vi "EndScript.vi"(8 "error in (no error)":errorcluster, 11 "VISA Refnum in":refnum<visa-resource-name>) -> (0 "error out":errorcluster, 2 "Tx for stopping code":string, 3 "VISA Refnum out":refnum<visa-resource-name>)   [LabVIEW 2017]
panel:
  out "Reply":string
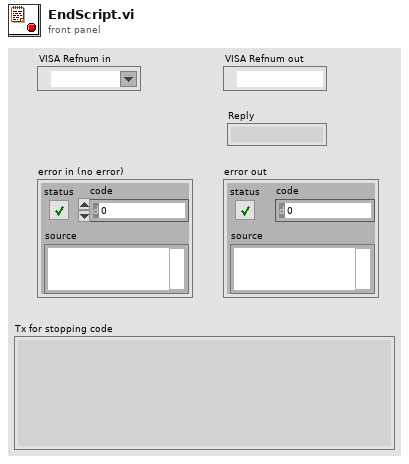
[diagram p1: front panel]
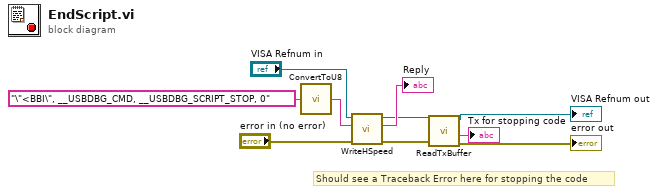
[diagram p0: block diagram]
diagram:
  # "Should see a Traceback Error here for stopping the code"
  n1 = call <userlib>:"ConvertToU8.vi"("struct"="\"<BBI\", __USBDBG_CMD, __USBDBG_SCRIPT_STOP, 0" ("write buffer")) -> ("Binary"=w6:string)
  n2 = call <userlib>:"WriteHSpeed.vi"("error in"="error in (no error)", "write buffer"=w6, "VISA Refnum in"="VISA Refnum in") -> ("error out"=w4:errorcluster, "read buffer"=→"Reply":string, "VISA Refnum out"=w3:refnum<visa-resource-name>)  [unwired: 6 in]
  n3 = call <userlib>:"ReadTxBuffer.vi"("error in"=w4, "VISA Refnum in"=w3) -> ("error out"=→"error out":errorcluster, "Tx Buffer"=→"Tx for stopping code":string, "VISA Refnum out"=→"VISA Refnum out":refnum<visa-resource-name>)  [unwired: 6 in, 1 out]
